vi "ScanivalveCollect.vi"(4 "error in (no error)":errorcluster, 6 "Samples per query.":i32=50, 7 "connection ID":refnum<k5>) -> (0 "error out":errorcluster, 1 "Tx Array":i16[][](array[numeric]), 2 "Px Array":sgl[][](array[numeric]), 3 "connection ID out":refnum<k5>)   [LabVIEW 2019]
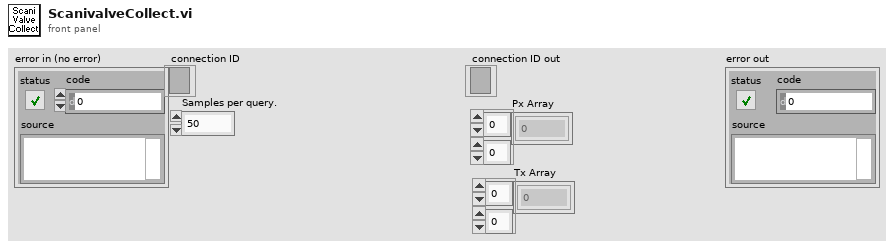
[diagram p1: front panel]
types:
  T1 = cluster{"Tx1":i16, "Tx2":i16, "Tx3":i16, "Tx4":i16, "Tx5":i16, "Tx6":i16, "Tx7":i16, "Tx8":i16, "Tx9":i16, "Tx10":i16, "Tx11":i16, "Tx12":i16, "Tx13":i16, "Tx14":i16, "Tx15":i16, "Tx16":i16}
  T2 = cluster{"Px1":sgl, "Px2":sgl, "Px3":sgl, "Px4":sgl, "Px5":sgl, "Px6":sgl, "Px7":sgl, "Px8":sgl, "Px9":sgl, "Px10":sgl, "Px11":sgl, "Px12":sgl, "Px13":sgl, "Px14":sgl, "Px15":sgl, "Px16":sgl}
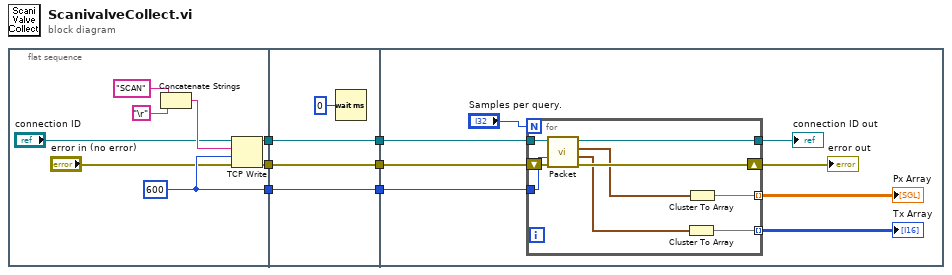
[diagram p0: block diagram]
diagram:
  n1 = flat-sequence {
    tunnel: [w11] -> w6
    tunnel: [w10] -> w5
    tunnel: [w9] -> w4
    tunnel: w6 -> [w18]
    tunnel: w5 -> [w17]
    tunnel: w4 -> [w16]
    tunnel: [w18] -> w3
    tunnel: [w17] -> w2
    tunnel: [w16] -> w1
    tunnel: w3 -> [w20]
    tunnel: w2 -> [w21]
    tunnel: w1 -> [w19]
    frame #0 {
      w9 = 600 ("timeout ms (25000)")
      n2 = Concatenate Strings("SCAN", "\r") -> (w12:string)
      n3 = TCP Write(connection ID="connection ID", data in=w12, error in (no error)="error in (no error)", 9:w9) -> (connection ID out=w10:refnum<k5>, error out=w11:errorcluster)  [unwired: 1 out]
    }
    frame #1 {
      n4 = Wait (ms)(milliseconds to wait=u32 0) -> ()  [unwired: 1 out]
    }
    frame #2 {
      n5 = for {
        N: "Samples per query." -> [_]
        tunnel: w21 -> [w34]
        tunnel: w19 -> [w33]
        tunnel: [w32] -> w23
        shift-right: [w31] -> w24
        shift-left: w20 -> [w35]
        tunnel: [w27] -> w26 mode=indexing
        tunnel: [w29] -> w25 mode=indexing
        n6 = call "Packet.vi"("error in (no error)"=w35, "timeout ms (10000)"=w33, "connection ID"=w34) -> ("error out"=w31:errorcluster, "tx"=w28:T1, "px"=w30:T2, "connection ID out"=w32:refnum<k5>)  [unwired: 3 in, 2 out]
        n7 = Cluster To Array(cluster=w28) -> (array=w27:i16[])
        n8 = Cluster To Array(cluster=w30) -> (array=w29:sgl[])
      }
      "connection ID out" <- w23
      "error out" <- w24
      "Px Array" <- w25
      "Tx Array" <- w26
    }
  }
